vi "RunDigitizer_nice.vi"() -> ()   [LabVIEW 2014]
doc: "Use this template to build a producer/consumer design pattern with events to produce queue items. Use this design pattern instead of the User Interface Event Handler pattern for user interfaces when you want to execute code asynchronously in response to an event without slowing the user interface responsiveness."
uses:
  <vilib>/addons/h5labview2/base/hid_t.ctl
  <vilib>/addons/h5labview2/base/lib_path.vi
  <vilib>/addons/h5labview2/base/H5Equery.vi
  <vilib>/addons/h5labview2/dataset/H5Dwrite.llb/H5Dwrite.xnode
  Program Files (x86)/CAEN/Comm/labview/CAENComm.lvlib
  <vilib>/addons/h5labview2/group/H5G.lvlib
panel:
  out "Wfm Plot 2":dbl[][](graph)
  out "TRIG_REC":u32
  out "Wfm Plot":dbl[][](graph)
  in  "VME Base Address 2":u32 format="%.0x"
  out "# Events Written":i32
  in  "# Events to\nRecord":i32
  in  "VME Base Address":u32 format="%.0x"
  out "Acquisition\nErrors":errorcluster
  out "Analysis\nErrors":errorcluster
  in  "Calibrate Verniers":bool
  in  "Stop Acquisition":bool
  in  "Start Acquisition":bool
  in  "Configure Output":bool
  in  "Calibrate Pedestals":bool
  in  "stop":bool
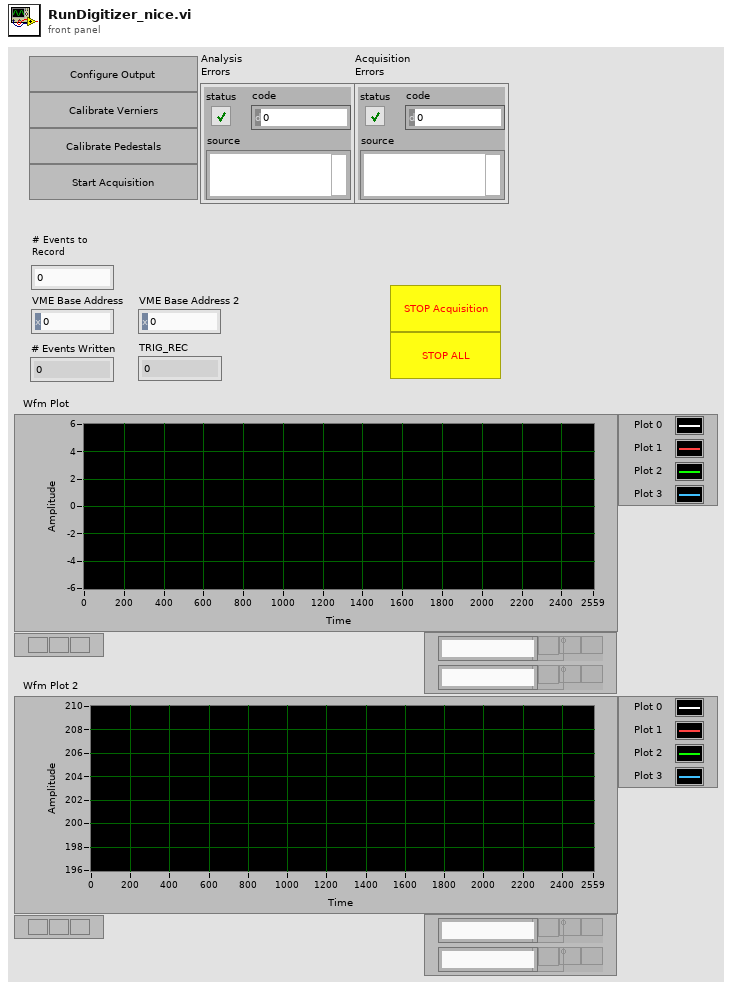
[diagram p1: front panel]
types:
  T1 = typedef "hid_t.ctl" = i32
  T2 = cluster{"State":enum16{"Startup", "Initialise", "Event OK", "Discard Event", "Exit", "Close"}, "Data":variant}
  T3 = enum16{"Configure", "Initialise", "Run", "Close"}
  T4 = enum16{"Startup", "Initialise", "Event OK", "Discard Event", "Exit", "Close"}
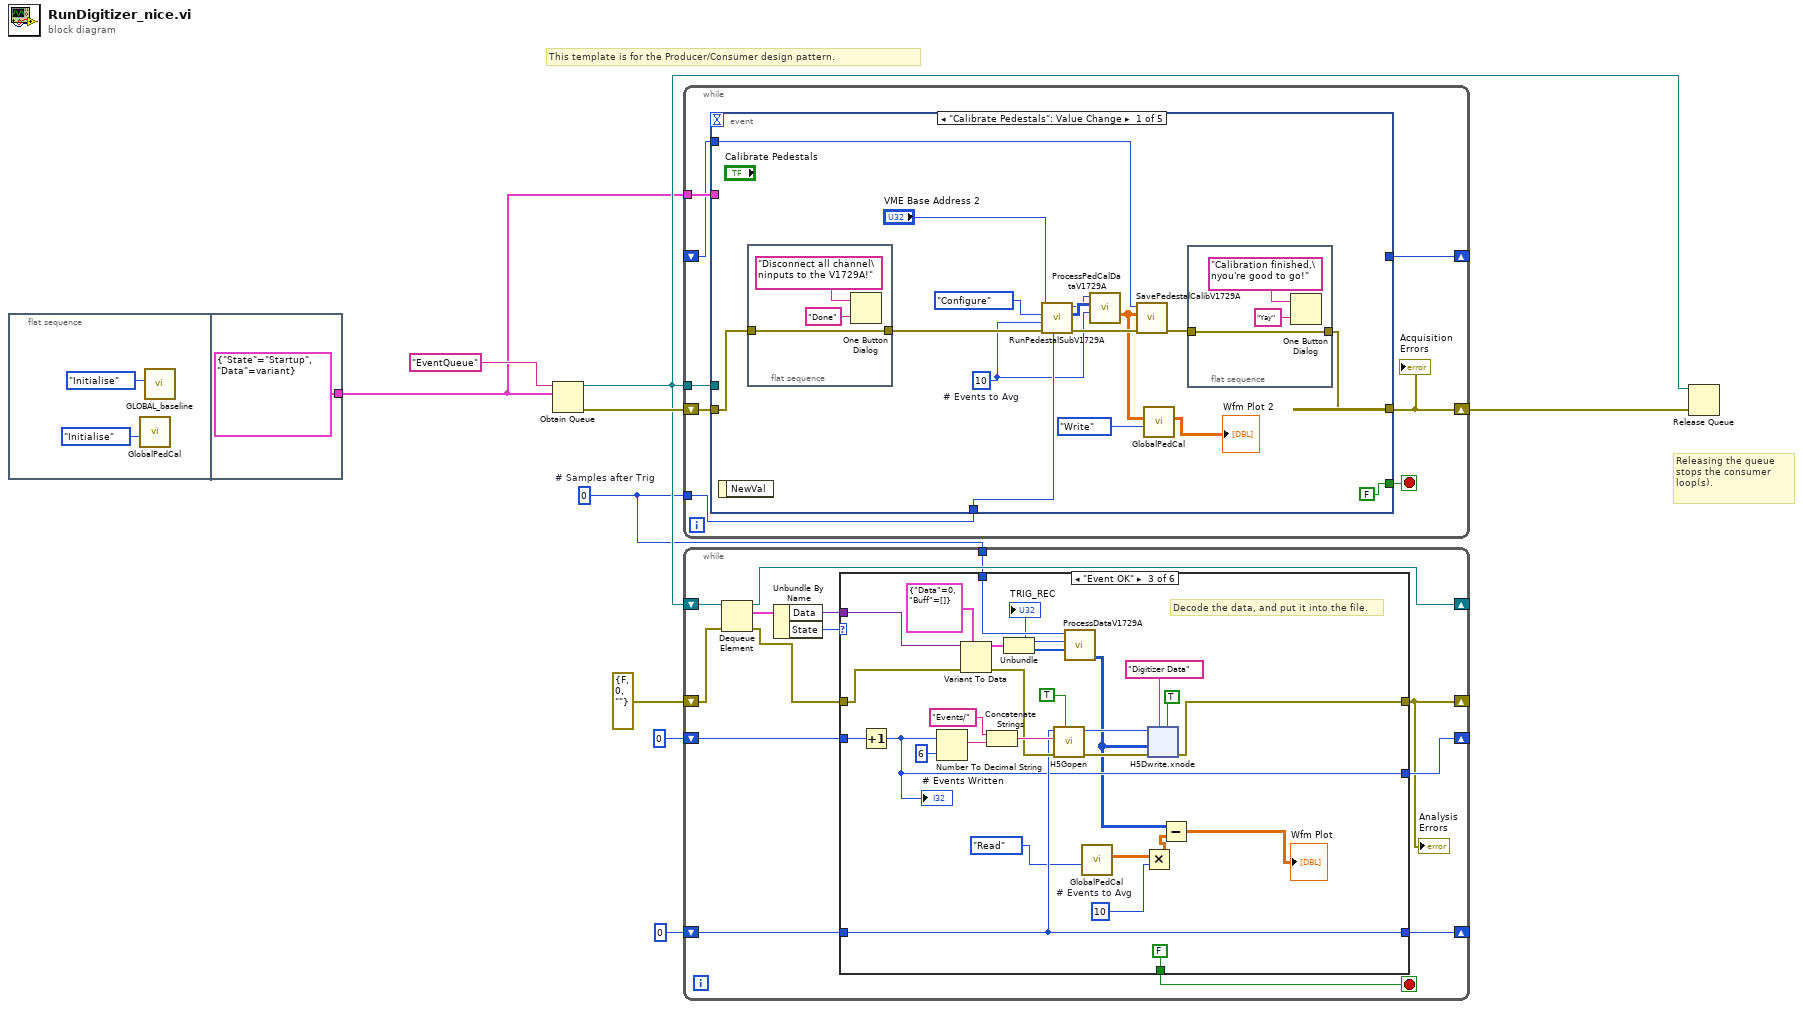
[diagram p0: block diagram]
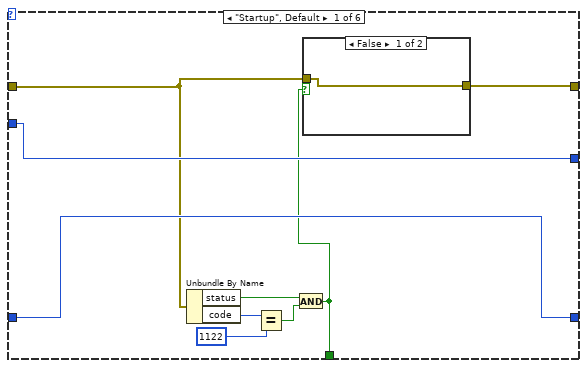
[diagram p2: hidden frame]
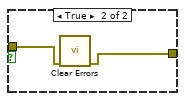
[diagram p3: hidden frame]
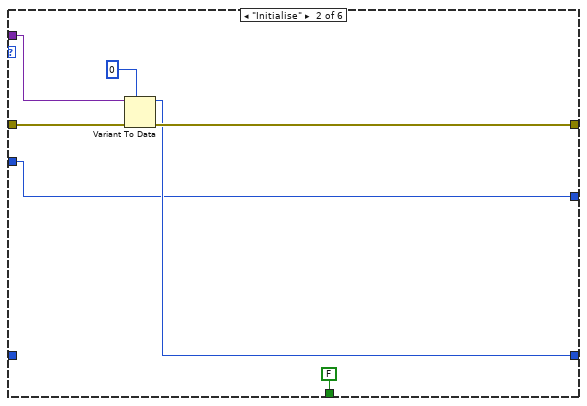
[diagram p4: hidden frame]
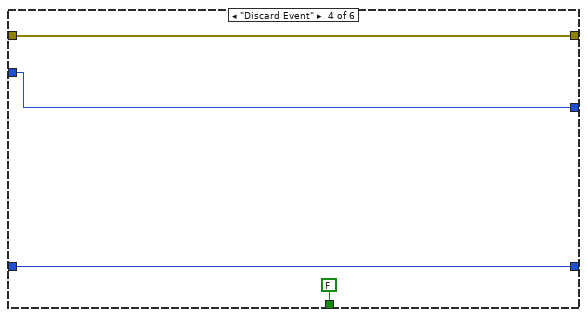
[diagram p5: hidden frame]
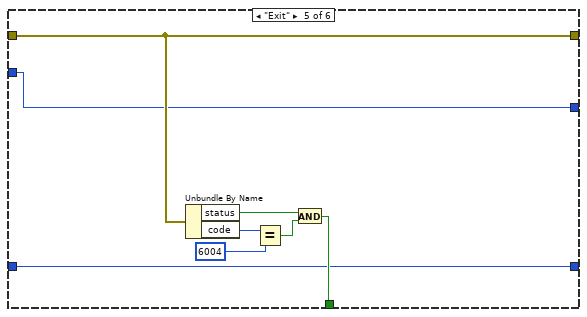
[diagram p6: hidden frame]
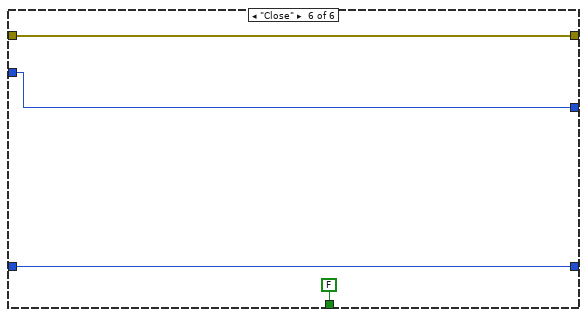
[diagram p7: hidden frame]
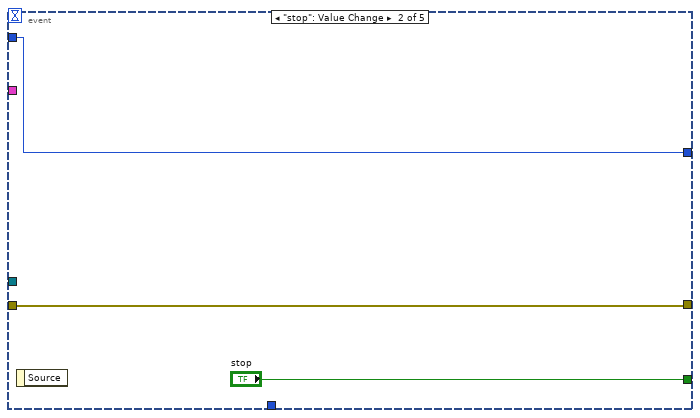
[diagram p8: hidden frame]
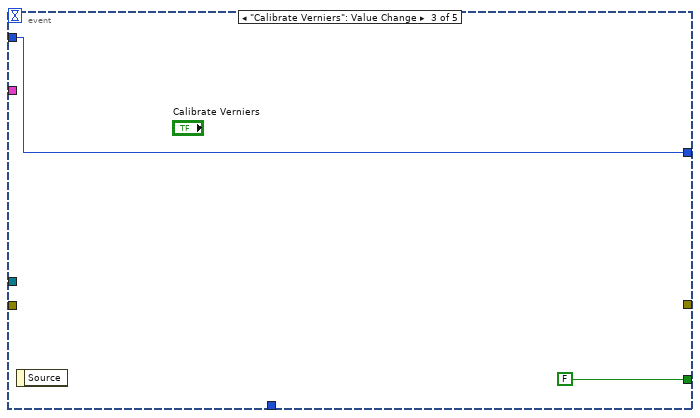
[diagram p9: hidden frame]
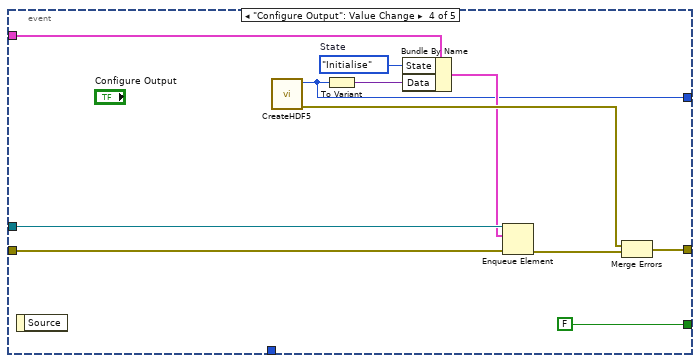
[diagram p10: hidden frame]
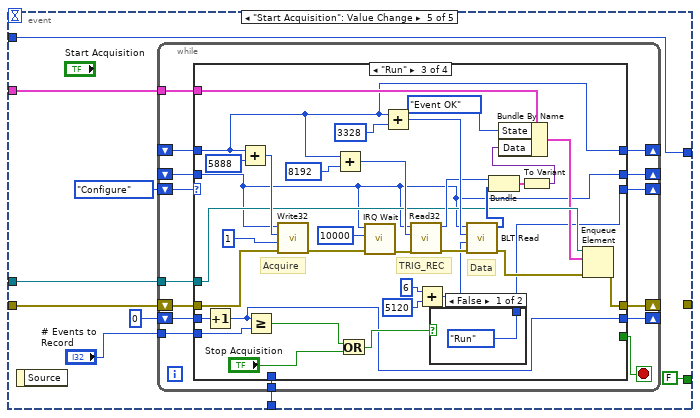
[diagram p11: hidden frame]
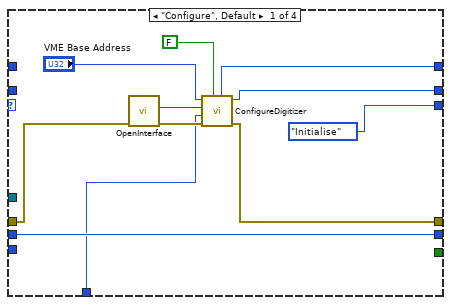
[diagram p12: hidden frame]
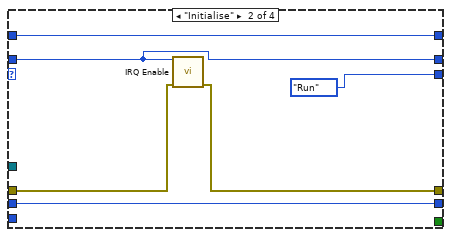
[diagram p13: hidden frame]
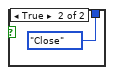
[diagram p14: hidden frame]
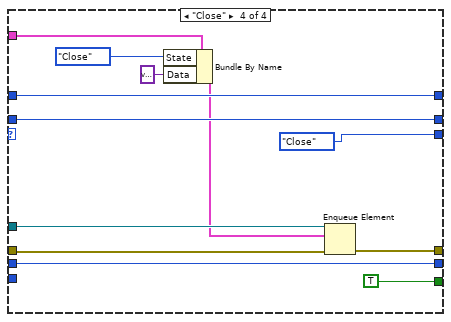
[diagram p15: hidden frame]
diagram:
  w1 = u16 0  # # Samples after Trig
  # "Releasing the queue stops the consumer loop(s)."
  # "This template is for the Producer/Consumer design pattern."
  n1 = flat-sequence {
    tunnel: [T2 {"State"=enum."Startup", "Data"=variant}] -> w2
    frame #0 {
      n2 = call "GlobalPedCal.vi"("State"=enum16{"Initialise", "Write", "Read"}."Initialise") -> ()  [unwired: 10 in, 1 out]
      n3 = call "GLOBAL_baseline.vi"("State"=enum16{"Initialise", "Write", "Read"}."Initialise") -> ()  [unwired: 10 in, 1 out]
    }
    frame #1 {
    }
  }
  n4 = Obtain Queue(name (unnamed)="EventQueue", element data type=w2) -> (queue out=w4:refnum<queue>, error out=w9:errorcluster)  [unwired: 3 in, 1 out]
  n5 = while {
    shift-right: [w18] -> w6
    shift-left: w9 -> [w19]
    tunnel: w4 -> [w20]
    tunnel: w2 -> [w16]
    tunnel: w1 -> [w15]
    shift-right: [w14] -> _
    shift-left: _ -> [w13]
    stop <- w17 stop-if-true
    n6 = event shown="[0] \"Calibrate Pedestals\": Value Change" {
      selector: _ -> [_ _ _ _ _]
      dyn-events: _ -> [_ _ _ _ _]
      timeout: _ -> [_ _ _ _ _]
      tunnel: w20 -> [_ _ _ w50 w63]
      tunnel: w19 -> [w30 w44 _ w51 w65]
      tunnel: [w27 w44 _ w54 _] -> w18
      tunnel: [FALSE ("stop") "stop" FALSE ("stop") FALSE ("stop") FALSE ("stop")] -> w17
      tunnel: w16 -> [_ _ _ w55 w64]
      tunnel: w15 -> [w35 _ _ _ w60]
      tunnel: [_ w43 w46 w48 w59] -> w14
      tunnel: w13 -> [w31 w43 w46 _ w59]
      event "Calibrate Pedestals": Value Change {
        w26 = 10  # # Events to Avg
        n7 = event-data() -> ()  [unwired: 1 in, 1 out]
        n8 = flat-sequence {
          tunnel: w30 -> [w42]
          tunnel: [w42] -> w29
          frame #0 {
            n9 = One Button Dialog(message="Disconnect all channel\ninputs to the V1729A!", button name ("OK")="Done") -> ()  [unwired: 1 out]
          }
        }
        n10 = call "RunPedestalSubV1729A.vi"("# Samples after Trig"=w35, "error in (no error)"=w29, "handle in"=w26, "Init State"=T3."Configure", "VME Base Address in"="VME Base Address 2") -> ("error out"=w34:errorcluster, "Data Out"=w25:u32[][], "Offset"=w22:i16)  [unwired: 3 in, 1 out]
        n11 = call "ProcessPedCalDataV1729A.vi"("# Events to Avg"=w26, "Data In"=w25, "Offset"=w22) -> ("Channel Data"=w24:dbl[][])  [unwired: 8 in]
        n12 = call "SavePedestalCalibV1729A.vi"("error in (no error)"=w34, "Data In"=w24, "File Handle"=w31) -> ("error out"=w28:errorcluster)  [unwired: 8 in]
        n13 = call "GlobalPedCal.vi"("State"=enum16{"Initialise", "Write", "Read"}."Write", "Data In"=w24) -> ("Data Out"=→"Wfm Plot 2":dbl[][])  [unwired: 9 in]
        n14 = flat-sequence {
          tunnel: w28 -> [w39]
          tunnel: [w39] -> w27
          frame #0 {
            n15 = One Button Dialog(message="Calibration finished,\nyou're good to go!", button name ("OK")="Yay") -> ()  [unwired: 1 out]
          }
        }
      }
      event "stop": Value Change {
        n16 = event-data() -> ()  [unwired: 1 in, 1 out]
      }
      event "Calibrate Verniers": Value Change {
        n17 = event-data() -> ()  [unwired: 1 in, 1 out]
      }
      event "Configure Output": Value Change {
        w56 = T4."Initialise"  # State
        n18 = event-data() -> ()  [unwired: 1 in, 1 out]
        n19 = call "CreateHDF5.vi"() -> ("error out"=w53:errorcluster, "File Handle"=w48:T1)  [unwired: 10 in]
        n20 = To Variant(anything=w48) -> (Variant=w57:variant)
        n21 = Bundle By Name(cluster=w55, "State"=w56, "Data"=w57) -> (w49:T2)
        n22 = Enqueue Element(queue=w50, element=w49, error in (no error)=w51) -> (error out=w52:errorcluster)  [unwired: 1 in, 2 out]
        n23 = Merge Errors(w53, w52) -> (w54:errorcluster)
      }
      event "Start Acquisition": Value Change {
        n24 = event-data() -> ()  [unwired: 1 in, 1 out]
        n25 = while {
          shift-right: [w75] -> _
          shift-left: T3."Configure" -> [w82]
          shift-right: [w80] -> _
          shift-left: w65 -> [w81]
          shift-right: [w79] -> _
          shift-left: _ -> [w76]
          shift-right: [w78] -> _
          shift-left: _ -> [w77]
          tunnel: w64 -> [w74]
          tunnel: w63 -> [w73]
          tunnel: "# Events to\nRecord" -> [w71]
          shift-right: [w69] -> _
          shift-left: 0 -> [w72]
          tunnel: w60 -> [w68]
          stop <- w70 stop-if-true
          n26 = case shown="\"Run\"" w82 {
            tunnel: w81 -> [w93 w99 w128 w141]
            tunnel: [w90 w94 w109 w142] -> w80
            tunnel: [w87 w97 w102 w145] -> w79
            tunnel: [w86 w98 w101 w146] -> w78
            tunnel: w77 -> [_ w98 w101 w146]
            tunnel: w76 -> [_ w97 w102 w145]
            tunnel: [T3."Initialise" T3."Run" w106 T3."Close"] -> w75
            tunnel: w74 -> [_ _ w113 w137]
            tunnel: w73 -> [_ _ w112 w140]
            tunnel: w72 -> [w84 w95 w105 w143]
            tunnel: w71 -> [_ _ w104 _]
            tunnel: [_ _ _ TRUE] -> w70
            tunnel: [w84 w95 w100 w143] -> w69
            tunnel: w68 -> [w83 _ _ _]
            frame "Configure", Default {
              n27 = call "OpenInterface.vi"("error in (no error)"=w93) -> ("error out"=w92:errorcluster, "handle"=w91:i32)  [unwired: 8 in, 1 out]
              n28 = call "ConfigureDigitizer.vi"("Software Trig?"=FALSE, "error in (no error)"=w92, "# Samples after Trig"=w83, "handle"=w91, "VME Base Address"="VME Base Address") -> ("error out"=w90:errorcluster, "handle out"=w86:i32, "VME Base Address out"=w87:u32)  [unwired: 4 in]
            }
            frame "Initialise" {
              n29 = call "IRQ Enable.vi"("error in (no error)"=w99, "handle"=w98) -> ("error out"=w94:errorcluster)  [unwired: 9 in]
            }
            frame "Run" {
              # "Data"
              # "TRIG_REC"
              # "Acquire"
              n30 = Increment(x=w105) -> (x+1=w100:i32)
              n31 = Add(x=w102, y=u32 5888 ("x")) -> (x+y=w130:u32)
              n32 = Greater Or Equal?(x=w100, y=w104) -> (x >= y?=w103:bool)
              n33 = call "Write32.vi"("error in (no error)"=w128, "Data"=u32 1, "Address"=w130, "handle"=w101) -> ("error out"=w132:errorcluster)  [unwired: 7 in]
              n34 = Add(x=w102, y=u32 8192 ("x")) -> (x+y=w126:u32)
              n35 = Or(x=w103, y="Stop Acquisition") -> (x .or. y?=w107:bool)
              n36 = call "IRQ Wait.vi"("error in (no error)"=w132, "Timeout"=u32 10000, "handle"=w101) -> ("error out"=w125:errorcluster)  [unwired: 8 in]
              n37 = Add(x=w102, y=u32 3328 ("x")) -> (x+y=w122:u32)
              n38 = call "Read32.vi"("error in (no error)"=w125, "Address"=w126, "handle"=w101) -> ("error out"=w123:errorcluster, "Data"=w117:u32)  [unwired: 7 in]
              n39 = Add(x=6 ("BltSize"), y=5120 ("BltSize")) -> (x+y=w119:i32)
              n40 = case shown="False" w107 {
                tunnel: [T3."Run" T3."Close"] -> w106
                frame False {
                }
                frame True {
                }
              }
              n41 = call "BLT Read.vi"("error in (no error)"=w123, "BltSize"=w119, "Address"=w122, "handle"=w101) -> ("error out"=w110:errorcluster, "Buff"=w118:u32[])  [unwired: 5 in, 1 out]
              n42 = Bundle("Data"=w117, "Buff"=w118) -> (w116:cluster{"Data":u32, "Buff":u32[]})  [unwired: 1 in]
              n43 = To Variant(anything=w116) -> (Variant=w115:variant)
              n44 = Bundle By Name(cluster=w113, "State"=T4."Event OK", "Data"=w115) -> (w111:T2)
              n45 = Enqueue Element(queue=w112, element=w111, error in (no error)=w110) -> (error out=w109:errorcluster)  [unwired: 1 in, 2 out]
            }
            frame "Close" {
              n46 = Bundle By Name(cluster=w137, "State"=T4."Close", "Data"=variant) -> (w136:T2)
              n47 = Enqueue Element(queue=w140, element=w136, error in (no error)=w141) -> (error out=w142:errorcluster)  [unwired: 1 in, 2 out]
            }
          }
        }
      }
    }
    "Acquisition\nErrors" <- w18
  }
  n48 = while {
    shift-right: [w148] -> _
    shift-left: errorcluster {"status"=FALSE, "code"=0, "source"=""} ("error out") -> [w155]
    shift-right: [w156] -> _
    shift-left: w4 -> [w161]
    shift-right: [w153] -> _
    shift-left: T1 0 ("File Handle") -> [w152]
    tunnel: w1 -> [w151]
    shift-right: [w149] -> _
    shift-left: 0 -> [w150]
    stop <- w154 stop-if-true
    n49 = Dequeue Element(queue=w161, error in (no error)=w155) -> (queue out=w156:refnum<queue>, element=w160:T2, error out=w157:errorcluster)  [unwired: 1 in, 1 out]
    n50 = Unbundle By Name(w160) -> ("Data"=w158:variant, "State"=w159:T4)
    n51 = case shown="\"Event OK\"" w159 {
      tunnel: w158 -> [_ w178 w206 _ _ _]
      tunnel: w157 -> [w164 w177 w205 w230 w233 w242]
      tunnel: [w162 w176 w189 w230 w233 w242] -> w148
      tunnel: [w163 FALSE FALSE FALSE w234 FALSE] -> w154
      tunnel: [w166 w175 w188 w228 w232 w240] -> w153
      tunnel: w152 -> [w166 _ w188 w228 w232 w240]
      tunnel: w151 -> [_ _ w196 _ _ _]
      tunnel: w150 -> [w165 w174 w203 w227 w231 w239]
      tunnel: [w165 w174 w187 w227 w231 w239] -> w149
      frame "Startup", Default {
        n52 = Unbundle By Name(w164) -> ("status"=w170:bool, "code"=w168:i32)
        n53 = Equal?(x=w168, y=1122) -> (x = y?=w169:bool)
        n54 = And(x=w170, y=w169) -> (x .and. y?=w163:bool)
        n55 = case shown="False" w163 {
          tunnel: w164 -> [w171 w173]
          tunnel: [w171 w172] -> w162
          frame False {
          }
          frame True {
            n56 = call <vilib>:"Clear Errors.vi"("error in (no error)"=w173) -> ("error out"=w172:errorcluster)  [unwired: 5 in, 1 out]
          }
        }
      }
      frame "Initialise" {
        n57 = Variant To Data(error in=w177, type=T1 0 ("File Handle"), Variant=w178) -> (data=w175:T1, error out=w176:errorcluster)
      }
      frame "Event OK" {
        w181 = 10  # # Events to Avg
        # "Decode the data, and put it into the file."
        n58 = Increment(x=w203) -> (x+1=w187:i32)
        "# Events Written" <- w187
        n59 = Number To Decimal String(number=w187, width (-)=i16 6) -> (decimal integer string=w199:string)
        n60 = Variant To Data(error in=w205, type=cluster{"Data":u32, "Buff":u32[]} {"Data"=0, "Buff"=[]} ("output cluster"), Variant=w206) -> (data=w204:cluster{"Data":u32, "Buff":u32[]}, error out=w197:errorcluster)
        n61 = Concatenate Strings("Events/", w199) -> (w198:string)
        n62 = Unbundle(w204) -> ("Data"=w195:u32, "Buff"=w194:u32[])
        "TRIG_REC" <- w195
        n63 = call <vilib>:"H5Gopen.vi"("create? (F)"=TRUE, "error in (no error)"=w197, "name"=w198, "ref in"=w188) -> ("error out"=w190:errorcluster, "group out"=w191:T1)  [unwired: 6 in]
        n64 = call "ProcessDataV1729A.vi"("Buffer"=w194, "TRIG_REC"=w195, "# Samples after Trig"=w196) -> ("Channel Data"=w186:u16[][])  [unwired: 7 in, 1 out]
        n65 = call "GlobalPedCal.vi"("State"=enum16{"Initialise", "Write", "Read"}."Read") -> ("Data Out"=w184:dbl[][])  [unwired: 10 in]
        n66 = Multiply(x=w184, y=w181) -> (x*y=w183:dbl[][])
        n67 = xnode "H5Dwrite.xnode"("replace? (F)"=TRUE, "dataset name"="Digitizer Data", "error in (no error)"=w190, "data"=w186, "ref in"=w191) -> ("error out"=w189:errorcluster)  [unwired: 2 in, 2 out]
        n68 = Subtract(x=w186, y=w183) -> (x-y=→"Wfm Plot":dbl[][])
      }
      frame "Discard Event" {
      }
      frame "Exit" {
        n69 = Unbundle By Name(w233) -> ("status"=w238:bool, "code"=w236:i32)
        n70 = Equal?(x=w236, y=6004) -> (x = y?=w237:bool)
        n71 = And(x=w238, y=w237) -> (x .and. y?=w234:bool)
      }
      frame "Close" {
      }
    }
    "Analysis\nErrors" <- w148
  }
  n72 = Release Queue(queue=w4, error in (no error)=w6) -> ()  [unwired: 1 in, 3 out]
